vi "Create.vi"(8 "error in (no error)":errorcluster) -> (0 "error out":errorcluster, 3 "Model out":refnum<class "Model.lvclass">)   [LabVIEW 2020, in "Model.lvclass"]
uses:
  Model.lvclass
  Model.lvclass/Model.ctl
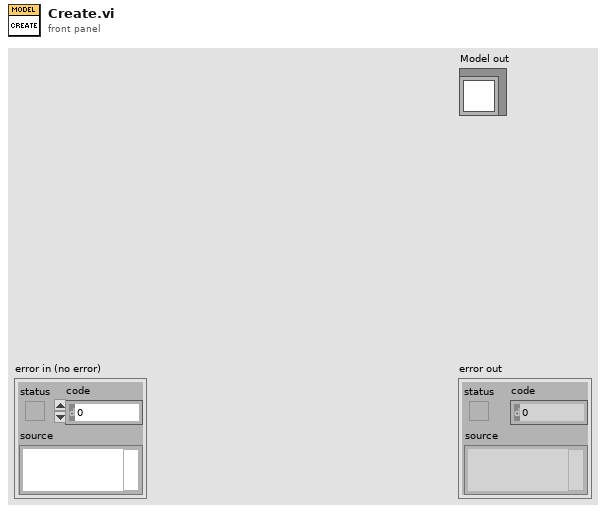
[diagram p1: front panel]
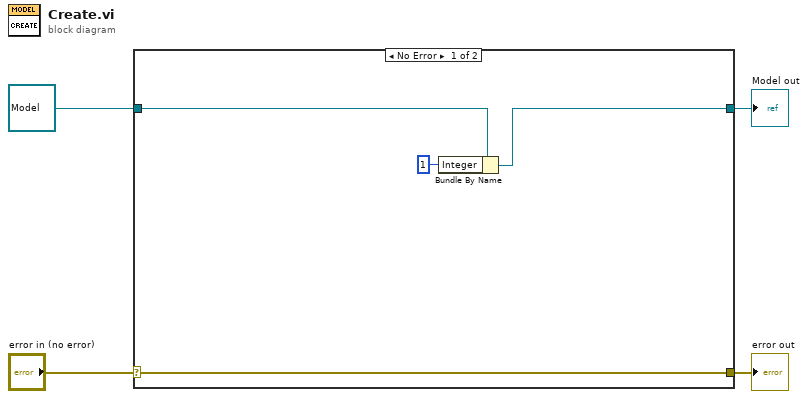
[diagram p0: block diagram]
diagram:
  n1 = case shown="No Error" "error in (no error)" {
    selector: "error in (no error)" -> [w8 w10]
    tunnel: [w8 w10] -> w3
    tunnel: [w5 w9] -> w2
    tunnel: refnum<class "Model.lvclass"> refnum ("Model in") -> [w7 w9]
    frame No Error {
      n2 = Bundle By Name(cluster=w7, "Integer"=1) -> (w5:refnum<class "Model.lvclass">)
    }
    frame Error {
    }
  }
  "error out" <- w3
  "Model out" <- w2
